vi "Invoke Network Endpoints Help.vi"   [LabVIEW 2020]
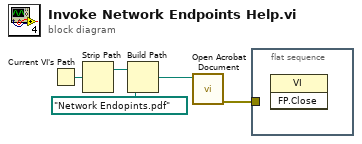
[diagram p0: block diagram]
diagram:
  n1 = Current VI's Path() -> (path=w1:path)
  n2 = Strip Path(path=w1) -> (stripped path=w2:path)  [unwired: 1 out]
  n3 = Build Path(base path=w2, name or relative path=path "Network Endopints.pdf") -> (appended path=w4:path)
  n4 = call <vilib>:"Open Acrobat Document.vi"("acrobat document"=w4) -> ("error out"=w3:errorcluster)  [unwired: 6 in]
  n5 = flat-sequence {
    tunnel: w3 -> [_]
    frame #0 {
      n6 = invoke class="VI" method="FP.Close"() -> ()  [unwired: 3 in, 3 out]
    }
  }
